vi "create available tags menu.vi"(9 "channel to map to":refnum<class "TBM channel.lvclass">, 10 "MenuRef":refnum<k9>, 11 "engine configuration in":refnum<class "engine configuration.lvclass">) -> (0 "error out":errorcluster)   [LabVIEW 2013, in "fixed channel tag bus module editor node.lvclass"]
uses:
  fixed channel tag bus module editor node.lvclass
  <vilib>/NI/Module Execution Interface/Engine Configuration/engine configuration.lvclass
  <vilib>/NI/Tag Bus Module Framework/channel/TBM channel.lvclass
  <vilib>/NI/Tag Bus/tag/tag descriptor.lvclass/tag descriptor.ctl
  <vilib>/NI/Tag Bus/tag/read tag name.vi
  <vilib>/NI/Tag Bus/tag/tag descriptor.lvclass
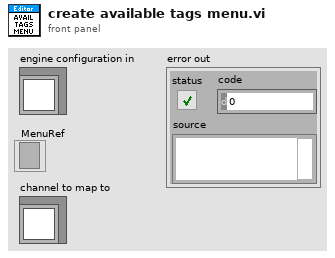
[diagram p1: front panel]
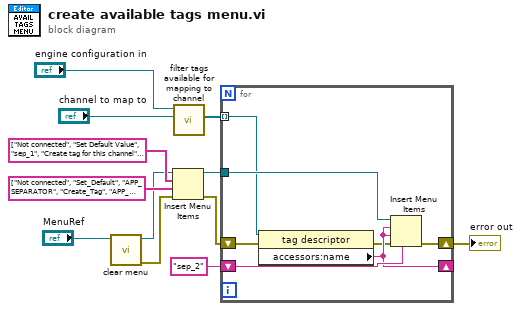
[diagram p0: block diagram]
diagram:
  n1 = call "clear menu.vi"("Menu in"="MenuRef") -> ("error out"=w4:errorcluster, "Menu out"=w8:refnum<k9>)  [unwired: 9 in]
  n2 = Insert Menu Items(6:w4, 7:string[] ["Not connected", "Set_Default", "APP_SEPARATOR", "Create_Tag", "APP_SEPARATOR"] ("item tags"), 8:string[] ["Not connected", "Set Default Value", "sep_1", "Create tag for this channel", "sep_2"] ("item names"), 9:w8) -> (0:w3:errorcluster, 3:w9:refnum<k9>)  [unwired: 2 in, 1 out]
  n3 = call <vilib>:"filter tags available for mapping to channel.vi"("channel to map to"="channel to map to", "engine configuration in"="engine configuration in") -> ("filtered tags"=w7:refnum<class "tag descriptor.lvclass">[])  [unwired: 8 in, 1 out]
  n4 = for {
    tunnel: w9 -> [w19]
    tunnel: w7 -> [w18] mode=indexing
    shift-right: [w16] -> _
    shift-left: "sep_2" -> [w17]
    shift-right: [w13] -> w2
    shift-left: w3 -> [w15]
    n5 = property class="tag descriptor"(reference=w18, error in=w15) -> (error out=w14:errorcluster, "accessors:name"=w16:string)  [unwired: 1 out]
    n6 = Insert Menu Items(4:w17, 6:w14, 7:w16, 8:w16, 9:w19) -> (0:w13:errorcluster)  [unwired: 1 in, 2 out]
  }
  "error out" <- w2
